vi "MultiChannel Write.vi"(8 "错误输入":cluster{"状态":bool, "代码":i32, "源":string}, 10 "数据至记录":dbl[][](array[numeric]), 11 "文件引用句柄输入":refnum<file>) -> (0 "错误输出":cluster{"状态":bool, "代码":i32, "源":string}, 3 "文件引用句柄输出":refnum<file>)   [LabVIEW 2012]
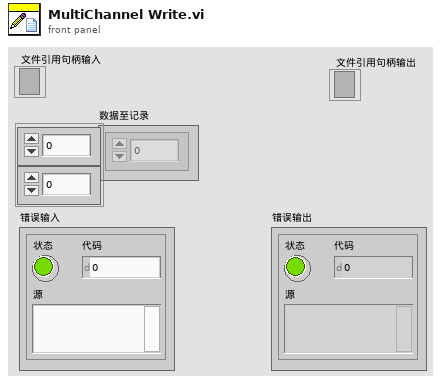
[diagram p1: front panel]
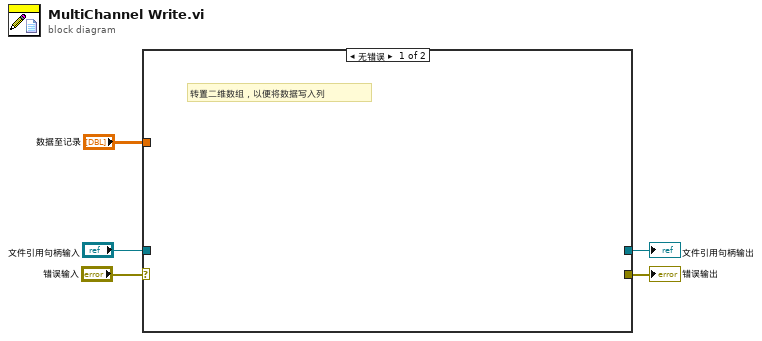
[diagram p0: block diagram]
diagram:
  n1 = case shown="无错误" "错误输入" {
    selector: "错误输入" -> [_ w7]
    tunnel: "文件引用句柄输入" -> [_ w6]
    tunnel: [_ w6] -> w3
    tunnel: [_ w7] -> w2
    tunnel: "数据至记录" -> [_ _]
    frame No Error {
      # "转置二维数组，以便将数据写入列"
    }
    frame Error {
    }
  }
  "错误输出" <- w2
  "文件引用句柄输出" <- w3
